vi "ELYSE_clock_pulses.vi"(6 "pulses previous":dbl, 8 "error in (no error)":errorcluster, 9 "ControlQueue":refnum<queue>, 10 "divider":dbl, 11 "DAQmxTaksContainer_General in":refnum<class "DAQmxTaksContainer_General.lvclass">) -> (0 "error out":errorcluster, 2 "pulses":dbl, 3 "DAQmxTaksContainer_General out":refnum<class "DAQmxTaksContainer_General.lvclass">)   [LabVIEW 2015, in "DAQmxTaksContainer_General.lvclass"]
uses:
  DAQmxTaksContainer_General.lvclass
  DAQmxTaksContainer_General.lvclass/DAQmxTaksContainer_General.ctl
  dependecies/ControlsVIs/Clusters-def/DAQmx-ELYSE_pulse_counter.ctl
  dependecies/ControlsVIs/Clusters-def/Standard Command.ctl
  dependecies/ControlsVIs/Clusters-def/SERVER-Commands.ctl
  DAQmxTask.lvclass
  Control/Control-Server/Control-Server.lvclass
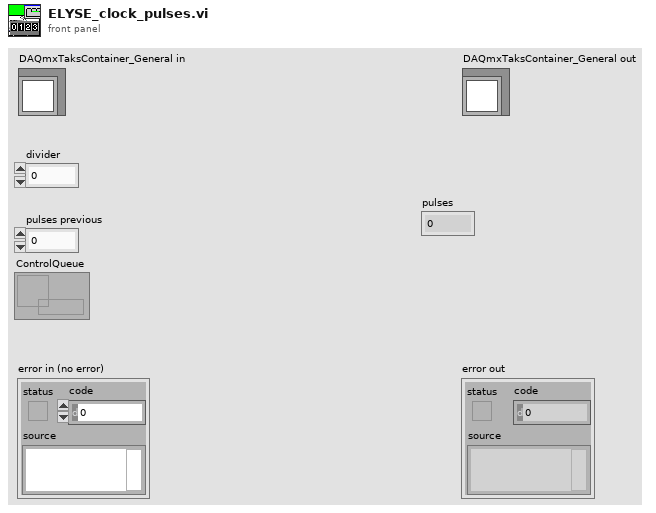
[diagram p1: front panel]
types:
  T1 = typedef "DAQmxTaksContainer_General.lvclass/DAQmx-ELYSE_pulse_counter.ctl" = cluster{"# counts":dbl}
  T2 = typedef "Standard Command.ctl" = cluster{"command":string, "data":variant}
  T3 = typedef "Control-Server.lvclass/SERVER-Commands.ctl" = string
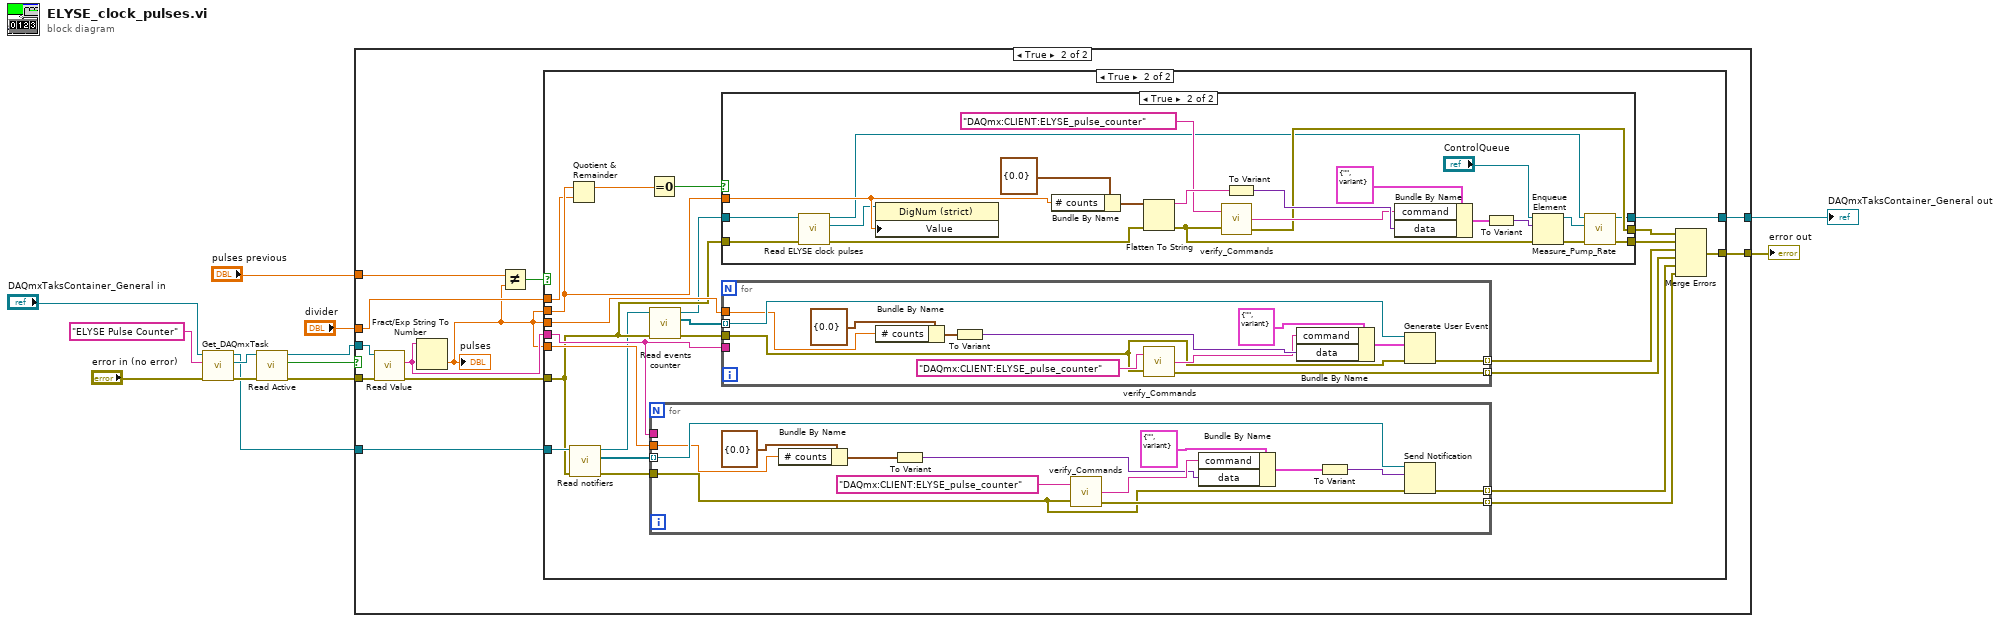
[diagram p0: block diagram]
diagram:
  n1 = call "Get_DAQmxTask.vi"("error in (no error)"="error in (no error)", "Task name"="ELYSE Pulse Counter", "DAQmxTaksContainer_General in"="DAQmxTaksContainer_General in") -> ("error out"=w12:errorcluster, "DAQmx Task"=w9:refnum<class "DAQmxTask.lvclass">, "DAQmxTaksContainer_General out"=w7:refnum<class "DAQmxTaksContainer_General.lvclass">)  [unwired: 6 in]
  n2 = call-dynamic "Read Active.vi"("error in (no error)"=w12, "DAQmxTask in"=w9) -> ("error out"=w11:errorcluster, "Active?"=w10:bool, "DAQmxTask out"=w8:refnum<class "DAQmxTask.lvclass">)  [unwired: 7 in]
  n3 = case shown="True" w10 {
    tunnel: w7 -> [w14 w17]
    tunnel: w11 -> [w15 w26]
    tunnel: w8 -> [_ w25]
    tunnel: [w14 w16] -> w6
    tunnel: [w15 w24] -> w5
    tunnel: "pulses previous" -> [_ w20]
    tunnel: "divider" -> [_ w19]
    frame False {
    }
    frame True {
      n4 = call-dynamic "Read Value.vi"("error in (no error)"=w26, "DAQmxTask en entrée"=w25) -> ("error out"=w23:errorcluster, "Data string"=w22:string)  [unwired: 6 in, 2 out]
      n5 = Fract/Exp String To Number(string=w22) -> (number=w18:dbl)  [unwired: 3 in, 1 out]
      "pulses" <- w18
      n6 = Not Equal?(x=w20, y=w18) -> (x != y?=w21:bool)
      n7 = case shown="True" w21 {
        tunnel: [w28 w47] -> w24
        tunnel: w23 -> [w28 w32]
        tunnel: w17 -> [w27 w33]
        tunnel: w22 -> [_ w40]
        tunnel: w18 -> [_ w37]
        tunnel: w19 -> [_ w36]
        tunnel: w18 -> [_ w35]
        tunnel: w18 -> [_ w34]
        tunnel: [w27 w29] -> w16
        frame False {
        }
        frame True {
          n8 = Quotient & Remainder(x=w37, y=w36) -> (x-y*floor(x/y)=w51:dbl)  [unwired: 1 out]
          n9 = call "Read notifiers.vi"("error in (no error)"=w32, "DAQmxTaksContainer_General in"=w33) -> ("error out"=w42:errorcluster, "notifiers"=w41:refnum<notifier>[], "DAQmxTaksContainer_General out"=w30:refnum<class "DAQmxTaksContainer_General.lvclass">)  [unwired: 7 in]
          n10 = Equal To 0?(x=w51) -> (x = 0?=w50:bool)
          n11 = call "Read events counter.vi"("error in (no error)"=w32, "DAQmxTaksContainer_General in"=w30) -> ("error out"=w46:errorcluster, "events counter"=w49:refnum<user-event>[], "DAQmxTaksContainer_General out"=w31:refnum<class "DAQmxTaksContainer_General.lvclass">)  [unwired: 7 in]
          n12 = for {
            tunnel: w42 -> [w54]
            tunnel: w41 -> [w57] mode=indexing
            tunnel: w40 -> [_]
            tunnel: [w58] -> w38 mode=indexing
            tunnel: [w53] -> w39 mode=indexing
            tunnel: w34 -> [w52]
            n13 = Bundle By Name(cluster=T1 {"# counts"=0.0} ("OSc:Read"), "# counts"=w52) -> (w61:T1)
            n14 = To Variant(anything=w61) -> (Variant=w62:variant)
            n15 = call "verify_Commands.vi"("Command"="DAQmx:CLIENT:ELYSE_pulse_counter" ("command"), "error in"=w54) -> ("Command out"=w64:string, "error out"=w58:errorcluster)  [unwired: 1 out]
            n16 = Bundle By Name(cluster=T2 {"command"="", "data"=variant} ("command"), "command"=w64, "data"=w62) -> (w56:T2)
            n17 = To Variant(anything=w56) -> (Variant=w55:variant)
            n18 = Send Notification(notification=w55, notifier=w57, error in (no error)=w54) -> (error out=w53:errorcluster)  [unwired: 1 out]
          }
          n19 = case shown="True" w50 {
            tunnel: w37 -> [_ w99]
            tunnel: w32 -> [w78 w85]
            tunnel: [w78 w82] -> w45
            tunnel: [_ w89] -> w44
            tunnel: w31 -> [w77 w86]
            tunnel: [w77 w80] -> w29
            frame False {
            }
            frame True {
              n20 = call "Read ELYSE clock pulses.vi"("error in (no error)"=w85, "DAQmxTaksContainer_General in"=w86) -> ("error out"=w87:errorcluster, "ELYSE clock pulses"=w84:refnum<vi>, "DAQmxTaksContainer_General out"=w81:refnum<class "DAQmxTaksContainer_General.lvclass">)  [unwired: 7 in]
              n21 = property class="DigNum (strict)"(reference=w84, "Value"=w99) -> ()  [unwired: 1 in, 2 out]
              n22 = Bundle By Name(cluster=T1 {"# counts"=0.0} ("OSc:Read"), "# counts"=w99) -> (w93:T1)
              n23 = Flatten To String(anything=w93, error in (no error)=w87) -> (data string=w96:string, error out=w90:errorcluster)  [unwired: 2 in, 1 out]
              n24 = call "verify_Commands.vi"("Command"=T3 "DAQmx:CLIENT:ELYSE_pulse_counter" ("Commands"), "error in"=w90) -> ("Command out"=w91:string, "error out"=w89:errorcluster)  [unwired: 1 out]
              n25 = To Variant(anything=w96) -> (Variant=w95:variant)
              n26 = Bundle By Name(cluster=T2 {"command"="", "data"=variant} ("input cluster"), "command"=w91, "data"=w95) -> (w94:T2)
              n27 = To Variant(anything=w94) -> (Variant=w98:variant)
              n28 = Enqueue Element(queue="ControlQueue", element=w98, error in (no error)=w90) -> (queue out=w79:refnum<queue>, error out=w83:errorcluster)  [unwired: 1 in, 1 out]
              n29 = call "Measure_Pump_Rate.vi"("error in (no error)"=w83, "ControlQueue"=w79, "DAQmxTaksContainer_General in"=w81) -> ("error out"=w82:errorcluster, "DAQmxTaksContainer_General out"=w80:refnum<class "DAQmxTaksContainer_General.lvclass">)  [unwired: 7 in]
            }
          }
          n30 = for {
            tunnel: w40 -> [_]
            tunnel: w46 -> [w67]
            tunnel: w49 -> [w73] mode=indexing
            tunnel: [w72] -> w48 mode=indexing
            tunnel: [w66] -> w43 mode=indexing
            tunnel: w35 -> [w65]
            n31 = Bundle By Name(cluster=T1 {"# counts"=0.0} ("OSc:Read"), "# counts"=w65) -> (w71:T1)
            n32 = To Variant(anything=w71) -> (Variant=w70:variant)
            n33 = call "verify_Commands.vi"("Command"="DAQmx:CLIENT:ELYSE_pulse_counter" ("command"), "error in"=w67) -> ("Command out"=w68:string, "error out"=w66:errorcluster)  [unwired: 1 out]
            n34 = Bundle By Name(cluster=T2 {"command"="", "data"=variant} ("command"), "command"=w68, "data"=w70) -> (w75:T2)
            n35 = Generate User Event(user event=w73, event data cluster=w75, error in=w67) -> (error out=w72:errorcluster)  [unwired: 1 in, 1 out]
          }
          n36 = Merge Errors(w44, w45, w48, w43, w39, w38) -> (w47:errorcluster)
        }
      }
    }
  }
  "error out" <- w5
  "DAQmxTaksContainer_General out" <- w6
